vi "UDMA_READ_RAM.vi"(0 "TCP Network Connection in":refnum<k5>, 1 "BASE ADDR":u32=100, 2 "LENGTH":u32=100, 3 "INCREMENT":u32=100, 5 "error in (no error)":errorcluster) -> (14 "TCP Network Connection out":refnum<k5>, 16 "Oscilloscope":u32[](graph), 18 "Status":u8[](array[numeric]), 19 "error out":errorcluster)   [LabVIEW 2019]
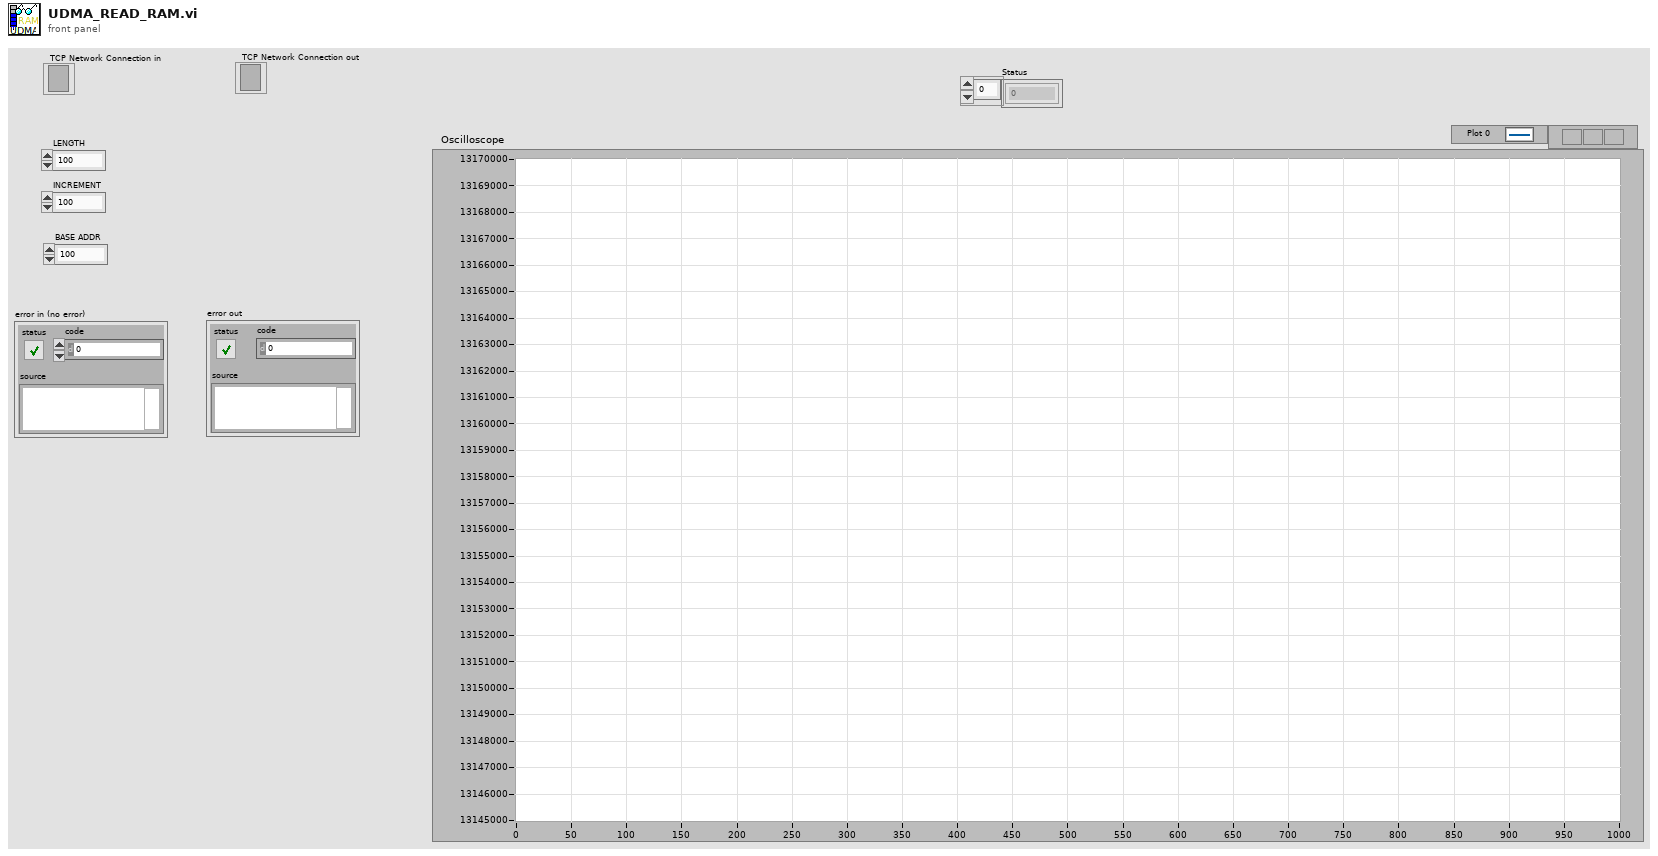
[diagram p1: front panel]
types:
  T1 = enum16{"big-endian, network order", "native, host order", "little-endian"}
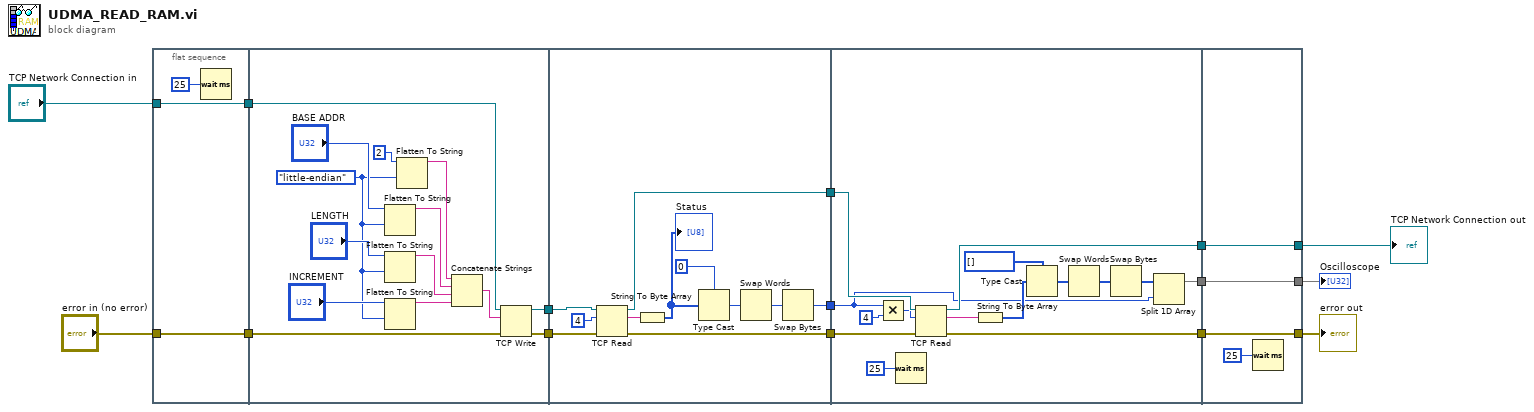
[diagram p0: block diagram]
diagram:
  n1 = flat-sequence {
    tunnel: [w17] -> w11
    tunnel: [w18] -> w10
    tunnel: "error in (no error)" -> [w18]
    tunnel: "TCP Network Connection in" -> [w17]
    tunnel: w11 -> [w32]
    tunnel: w10 -> [w31]
    tunnel: [w30] -> w5
    tunnel: [w29] -> w4
    tunnel: w5 -> [w40]
    tunnel: w4 -> [w43]
    tunnel: [w42] -> w3
    tunnel: [w33] -> w2
    tunnel: [w41] -> w1
    tunnel: w3 -> [w57]
    tunnel: w2 -> [w45]
    tunnel: [w56] -> w8
    tunnel: [w55] -> w7
    tunnel: [w46] -> w6
    tunnel: w1 -> [w58]
    tunnel: [w60] -> w9
    tunnel: [w61] -> w13
    tunnel: [w62] -> w12
    tunnel: w8 -> [w62]
    tunnel: w7 -> [w61]
    tunnel: w6 -> [w60]
    frame #0 {
      n2 = Wait (ms)(milliseconds to wait=u32 25) -> ()  [unwired: 1 out]
    }
    frame #1 {
      w19 = T1."little-endian" ("byte order (0:big-endian, network order)")
      n3 = Flatten To String(anything="BASE ADDR", byte order (0:big-endian, network order)=w19) -> (data string=w28:string)  [unwired: 2 in, 2 out]
      n4 = Flatten To String(anything="LENGTH", byte order (0:big-endian, network order)=w19) -> (data string=w23:string)  [unwired: 2 in, 2 out]
      n5 = Flatten To String(anything="INCREMENT", byte order (0:big-endian, network order)=w19) -> (data string=w22:string)  [unwired: 2 in, 2 out]
      n6 = Flatten To String(anything=u32 2 ("element"), byte order (0:big-endian, network order)=w19) -> (data string=w26:string)  [unwired: 2 in, 2 out]
      n7 = Concatenate Strings(w26, w28, w23, w22) -> (w25:string)
      n8 = TCP Write(connection ID=w32, data in=w25, error in (no error)=w31) -> (connection ID out=w30:refnum<k5>, error out=w29:errorcluster)  [unwired: 1 in, 1 out]
    }
    frame #2 {
      n9 = TCP Read(connection ID=w40, bytes to read=4, error in (no error)=w43) -> (connection ID out=w41:refnum<k5>, data out=w39:string, error out=w42:errorcluster)  [unwired: 2 in]
      n10 = String To Byte Array(string=w39) -> (unsigned byte array=w37:u8[])
      "Status" <- w37
      n11 = Type Cast(type=u32 0 ("y"), x=w37) -> (*(type *) &x=w36:u32)
      n12 = Swap Words(1:w36) -> (0:w35:u32)
      n13 = Swap Bytes(anything=w35) -> (byte swapped=w33:u32)
    }
    frame #3 {
      n14 = Multiply(x=w45, y=u32 4) -> (x*y=w53:u32)
      n15 = Wait (ms)(milliseconds to wait=u32 25) -> ()  [unwired: 1 out]
      n16 = TCP Read(connection ID=w58, bytes to read=w53, error in (no error)=w57) -> (connection ID out=w56:refnum<k5>, data out=w44:string, error out=w55:errorcluster)  [unwired: 2 in]
      n17 = String To Byte Array(string=w44) -> (unsigned byte array=w51:u8[])
      n18 = Type Cast(type=u32[] [], x=w51) -> (*(type *) &x=w49:u32[])
      n19 = Swap Words(1:w49) -> (0:w48:u32[])
      n20 = Swap Bytes(anything=w48) -> (byte swapped=w47:u32[])
      n21 = Split 1D Array(array=w47, index=w45) -> (first subarray=w46:u32[])  [unwired: 1 out]
    }
    frame #4 {
      n22 = Wait (ms)(milliseconds to wait=u32 25) -> ()  [unwired: 1 out]
    }
  }
  "error out" <- w13
  "TCP Network Connection out" <- w12
  "Oscilloscope" <- w9
